vi "DispenseWait.vi"(8 "error in (no error)":errorcluster, 9 "delay":dbl, 10 "time":dbl, 11 "Ultimus V in":refnum<class "Ultimus V.lvclass">) -> (0 "error out":errorcluster, 3 "Ultimus V out":refnum<class "Ultimus V.lvclass">)   [LabVIEW 2020, in "Ultimus V.lvclass"]
uses:
  Ultimus V.lvclass
  Dispenser.lvclass
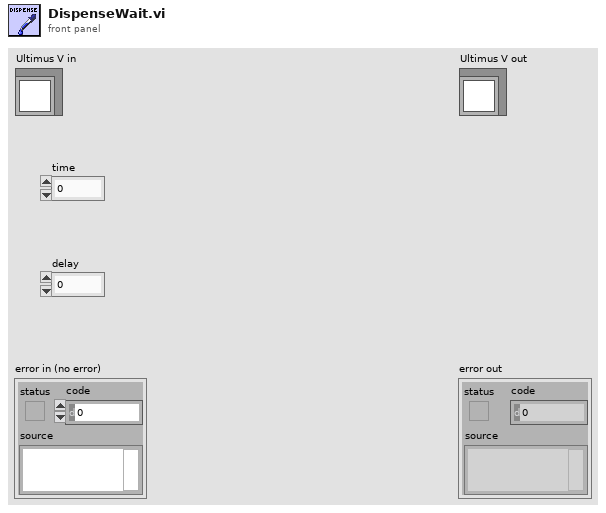
[diagram p1: front panel]
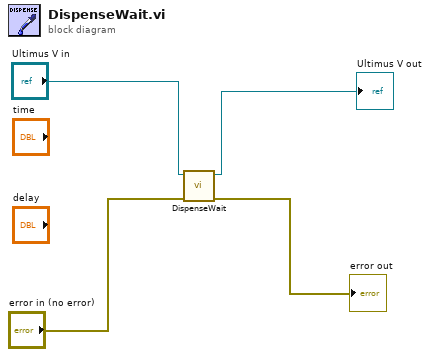
[diagram p0: block diagram]
diagram:
  n1 = call-parent "DispenseWait.vi"("error in (no error)"="error in (no error)", "Dispenser in"="Ultimus V in") -> ("error out"=→"error out":errorcluster, "Dispenser out"=→"Ultimus V out":refnum<class "Ultimus V.lvclass">)  [unwired: 8 in]
